vi "Laser 1 Set Wavelength L3.vi"() -> ()   [LabVIEW 2017]
uses:
  Typedefs/UI ctrl refs cluster.ctl
  Typedefs/Imaging Param ref.ctl
  Typedefs/Laser control knob.ctl
  Typedefs/Frame Size.ctl
  Typedefs/Plane Mode.ctl
  Typedefs/PMT control knob.ctl
  Typedefs/XY Stage_Move.ctl
  User Interface/Queue/Message Queue/Typedefs/All Message Queues.ctl
  User Interface/Queue/Message Queue/Typedefs/Message Cluster.ctl
  Typedefs/Logging queue element.ctl
  Typedefs/Imaging Protocols enum.ctl
  Typedefs/Acquired points count.ctl
panel:
  in  "Queues Cluster":T1
  in  "Error in":errorcluster caption="Error in (no error)"
  in  "UI elements cluster":T2
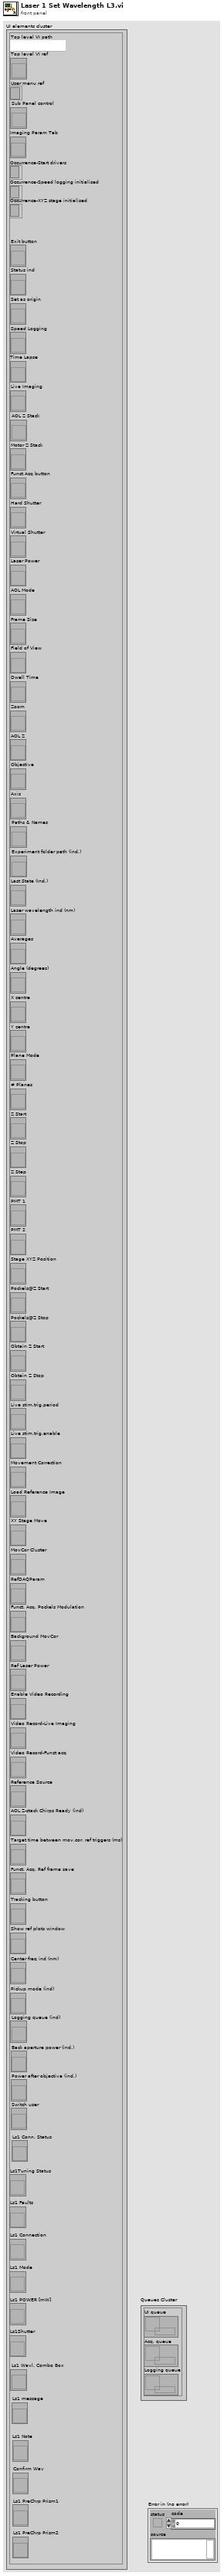
[diagram p1: front panel]
types:
  T1 = typedef "All Message Queues.ctl" = cluster{"UI queue":refnum<queue>, "Acq. queue":refnum<queue>, "Logging queue":refnum<queue>}
  T2 = typedef "UI ctrl refs cluster.ctl" = cluster{"Top level VI path":path, "Top level VI ref":refnum<vi>, "User menu ref":refnum<k9>, "Sub Panel control":refnum<vi>, "Imaging Param Tab":T3, "Occurrence-Start drivers":refnum<k4>, "Occurrence-Speed logging initialised":refnum<k4>, "Occurrence-XYZ stage initialised":refnum<k4>, "Exit button":refnum<vi>, "Status ind":refnum<vi>, "Set as origin":refnum<vi>, "Speed Logging":refnum<vi>, "Time Lapse":refnum<vi>, "Live Imaging":refnum<vi>, "AOL Z Stack":refnum<vi>, "Motor Z Stack":refnum<vi>, "Funct Acq button":refnum<vi>, "Hard Shutter":refnum<vi>, "Virtual Shutter":refnum<vi>, "Laser Power":refnum<vi>, "AOL Mode":refnum<vi>, "Frame Size":refnum<vi>, "Field of View":refnum<vi>, "Dwell Time":refnum<vi>, "Zoom":refnum<vi>, "AOL Z":refnum<vi>, "Objective":refnum<vi>, "Axis":refnum<vi>, "Paths & Names":refnum<vi>, "Experiment folder path (ind.)":refnum<vi>, "Last State (Ind.)":refnum<vi>, "Laser wavelength ind (nm)":refnum<vi>, "Averages":refnum<vi>, "Angle (degrees)":refnum<vi>, "X centre":refnum<vi>, "Y centre":refnum<vi>, "Plane Mode":refnum<vi>, "# Planes":refnum<vi>, "Z Start":refnum<vi>, "Z Stop":refnum<vi>, "Z Step":refnum<vi>, "PMT 1":refnum<vi>, "PMT 2":refnum<vi>, "Stage XYZ Position":refnum<vi>, "Pockels@Z Start":refnum<vi>, "Pockels@Z Stop":refnum<vi>, "Obtain Z Start":refnum<vi>, "Obtain Z Stop":refnum<vi>, "Live stim.trig.period":refnum<vi>, "Live stim.trig.enable":refnum<vi>, "Movement Correction":refnum<vi>, "Load Reference Image":refnum<vi>, "XY Stage Move":refnum<vi>, "MovCor Cluster":refnum<vi>, "RefDAQParam":refnum<vi>, "Funct. Acq. Pockels Modulation":refnum<vi>, "Background MovCor":refnum<vi>, "Ref Laser Power":refnum<vi>, "Enable Video Recording":refnum<vi>, "Video Record-Live Imaging":refnum<vi>, "Video Record-Funct acq":refnum<vi>, "Reference Source":refnum<vi>, "AOL Z-stack Chirps Ready (ind)":refnum<vi>, "Target time between mov.cor. ref triggers (ms)":refnum<vi>, "Funct. Acq. Ref frame save":refnum<vi>, "Tracking button":refnum<vi>, "Show ref plots window":refnum<vi>, "Center freq ind (nm)":refnum<vi>, "Pickup mode (ind)":refnum<vi>, "Logging queue (ind)":refnum<vi>, "Back aperture power (ind.)":refnum<vi>, "Power after objective (ind.)":refnum<vi>, "Switch user":refnum<vi>, "Ls1 Conn. Status":refnum<vi>, "Ls1Tuning Status":refnum<vi>, "Ls1 Faults":refnum<vi>, "Ls1 Connection":refnum<vi>, "Ls1 Mode":refnum<vi>, "Ls1 POWER [mW]":refnum<vi>, "Ls1Shutter":refnum<vi>, "Ls1 Wavl. Combo Box":refnum<vi>, "Ls1 message":refnum<vi>, "Ls1 Note":refnum<vi>, "Confirm Wav":refnum<vi>, "Ls1 PreChrp Prism1":refnum<vi>, "Ls1 PreChrp Prism2":refnum<vi>}
  T3 = typedef "Imaging Param ref.ctl" = refnum<vi>
  T4 = enum16{"Initialise Connections", "Initialise system", "Check Status", "Open/Close Shutter", "Set wavelength", "Close"}
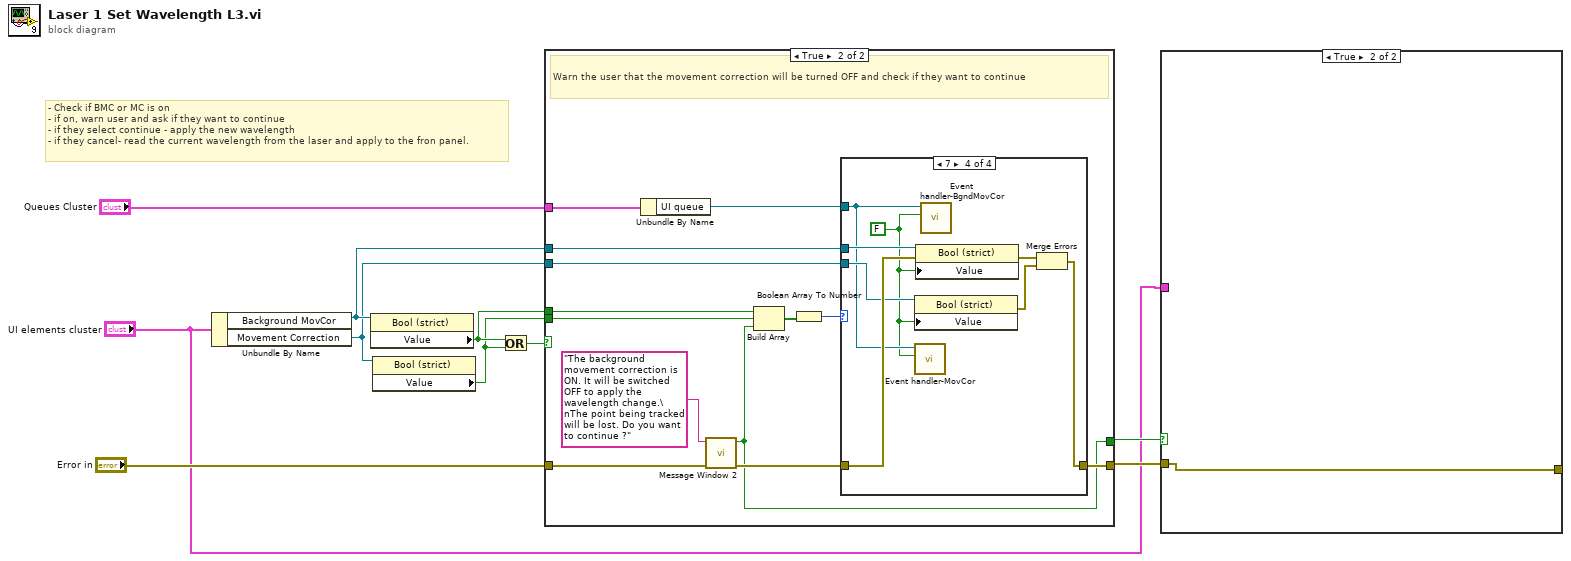
[diagram p0: block diagram]
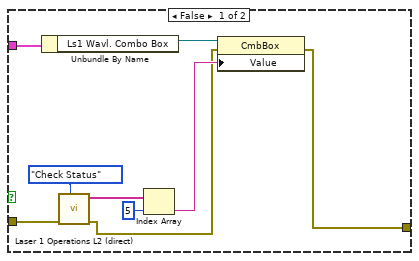
[diagram p2: hidden frame]
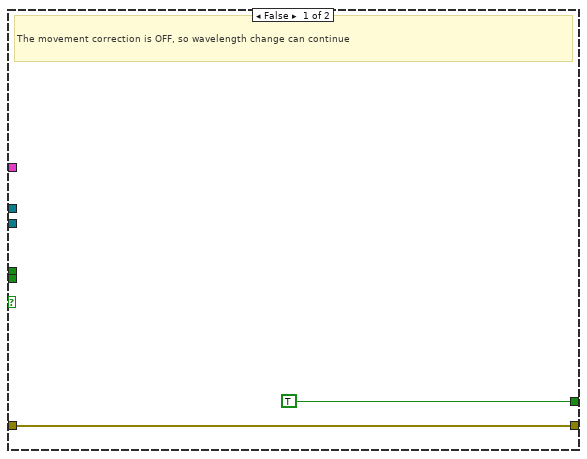
[diagram p3: hidden frame]
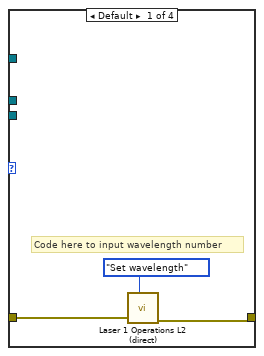
[diagram p4: hidden frame]
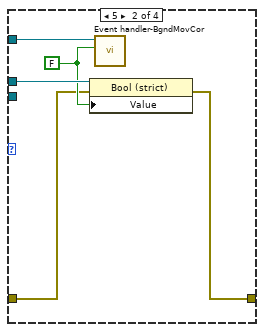
[diagram p5: hidden frame]
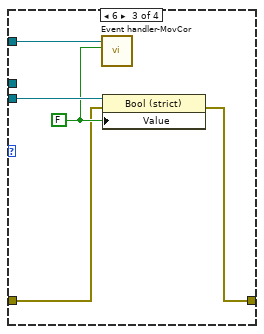
[diagram p6: hidden frame]
diagram:
  # "- Check if BMC or MC is on\n- if on, warn user and ask if they want to continue\n- if they select continue - apply the new wavelength\n- if they cancel- read the current wavelength from the laser and apply to the fron panel."
  n1 = Unbundle By Name("UI elements cluster") -> ("Background MovCor"=w4:refnum<vi>, "Movement Correction"=w3:refnum<vi>)
  n2 = property class="Bool (strict)"(reference=w4) -> ("Value"=w6:bool)  [unwired: 1 in, 2 out]
  n3 = property class="Bool (strict)"(reference=w3) -> ("Value"=w5:bool)  [unwired: 1 in, 2 out]
  n4 = Or(x=w6, y=w5) -> (x .or. y?=w10:bool)
  n5 = case shown="True" w10 {
    tunnel: "Error in" -> [w12 w25]
    tunnel: [w12 w14] -> w8
    tunnel: [TRUE ("Ok ?") w13] -> w7
    tunnel: "Queues Cluster" -> [_ w18]
    tunnel: w6 -> [_ w23]
    tunnel: w5 -> [_ w22]
    tunnel: w4 -> [_ w16]
    tunnel: w3 -> [_ w15]
    frame False {
      # "The movement correction is OFF, so wavelength change can continue"
    }
    frame True {
      # "Warn the user that the movement correction will be turned OFF and check if they want to continue"
      n6 = Unbundle By Name(w18) -> ("UI queue"=w17:refnum<queue>)
      n7 = call "Message Window 2.vi"("error in (no error)"=w25, "Message string"="The background movement correction is ON. It will be switched OFF to apply the wavelength change.\nThe point being tracked will be lost. Do you want to continue ?") -> ("error out (no error)"=w19:errorcluster, "Ok ?"=w13:bool)  [unwired: 8 in]
      n8 = Build Array(w23, w22, w13) -> (w21:bool[])
      n9 = Boolean Array To Number(Boolean array=w21) -> (number=w20:u32)
      n10 = case shown="7" w20 {
        tunnel: w19 -> [w28 w30 w35 w45]
        tunnel: w17 -> [_ w33 w38 w43]
        tunnel: w16 -> [_ w32 _ w46]
        tunnel: w15 -> [_ _ w37 w44]
        tunnel: [w27 w29 w34 w39] -> w14
        frame Default {
          # "Code here to input wavelength number"
          n11 = call "Laser 1 Operations L2 (direct).vi"("Laser Ops\n actions"=T4."Set wavelength" ("Laser Ops\n actions"), "error in (no error)"=w28) -> ("error out"=w27:errorcluster)  [unwired: 5 in, 4 out]
        }
        frame 5 {
          w31 = FALSE ("Background MovCor Button.NewVal")
          n12 = property class="Bool (strict)"(reference=w32, error in=w30, "Value"=w31) -> (error out=w29:errorcluster)  [unwired: 1 out]
          n13 = call "Event handler-BgndMovCor.vi"("Background MovCor Button.NewVal"=w31, "UI Queue"=w33) -> ()  [unwired: 10 in]
        }
        frame 6 {
          w36 = FALSE ("Value")
          n14 = call "Event handler-MovCor.vi"("Movement Correction ON?"=w36, "UI queue in"=w38) -> ()  [unwired: 9 in, 1 out]
          n15 = property class="Bool (strict)"(reference=w37, error in=w35, "Value"=w36) -> (error out=w34:errorcluster)  [unwired: 1 out]
        }
        frame 7 {
          w42 = FALSE ("Background MovCor Button.NewVal")
          n16 = property class="Bool (strict)"(reference=w44, "Value"=w42) -> (error out=w40:errorcluster)  [unwired: 1 in, 1 out]
          n17 = call "Event handler-MovCor.vi"("Movement Correction ON?"=w42, "UI queue in"=w43) -> ()  [unwired: 9 in, 1 out]
          n18 = property class="Bool (strict)"(reference=w46, error in=w45, "Value"=w42) -> (error out=w41:errorcluster)  [unwired: 1 out]
          n19 = call "Event handler-BgndMovCor.vi"("Background MovCor Button.NewVal"=w42, "UI Queue"=w43) -> ()  [unwired: 10 in]
          n20 = Merge Errors(w41, w40) -> (w39:errorcluster)
        }
      }
    }
  }
  n21 = case shown="True" w7 {
    tunnel: w8 -> [w55 w56]
    tunnel: "UI elements cluster" -> [w51 _]
    tunnel: [w47 w56] -> _
    frame False {
      n22 = Unbundle By Name(w51) -> ("Ls1 Wavl. Combo Box"=w50:refnum<vi>)
      n23 = call "Laser 1 Operations L2 (direct).vi"("Laser Ops\n actions"=T4."Check Status" ("Laser Ops\n actions"), "error in (no error)"=w55) -> ("error out"=w48:errorcluster, "Data"=w53:string[])  [unwired: 5 in, 3 out]
      n24 = Index Array(array=w53, index=5) -> (element=w49:string)
      n25 = property class="CmbBox"(reference=w50, error in=w48, "Value"=w49) -> (error out=w47:errorcluster)  [unwired: 1 out]
    }
    frame True {
    }
  }
